vi "SetCheckedStatus.vi"(8 "error in (no error)":errorcluster, 9 "Checked":bool, 10 "MenuItem":refnum<class "MGI_MenuItem.lvclass">, 11 "Control in":refnum<class "MGI_Control.lvclass">) -> (0 "error out":errorcluster, 3 "Control out":refnum<class "MGI_Control.lvclass">)   [LabVIEW 2016, in "MGI_Control.lvclass"]
doc: "Sets the Checked Status.\n\nAuthored by Derek E. Trepanier\nsupport@mooregoodideas.com\nwww.mooregoodideas.com\n\nCopyright (c) 2012, Moore Good Ideas, Inc.\n\nAll rights reserved.\n\nRedistribution and use in source and binary forms, with or without modification, are permitted provided that the following conditions are met:\n\n * Redistributions of source code must retain the above copyright notice, this list of conditions and the following disclaimer.\n * Redistributions in binary form must reproduce the above copyright notice, this list of conditions and the following disclaimer in the documentation and/or other materials provided with the distribution.\n * Neither the name of Moore Good Ideas, Inc. nor the names of its contributors may be used to endorse or promote products derived from this software without specific prior written permission.\n\nTHIS SOFTWARE IS PROVIDED BY THE COPYRIGHT HOLDERS AND CONTRIBUTORS \"AS IS\" AND ANY EXPRESS OR IMPLIED WARRANTIES, INCLUDING, BUT NOT LIMITED TO, THE IMPLIED WARRANTIES OF MERCHANTABILITY AND FITNESS FOR A PARTICULAR PURPOSE ARE DISCLAIMED. IN NO EVENT SHALL THE COPYRIGHT OWNER OR CONTRIBUTORS BE LIABLE FOR ANY DIRECT, INDIRECT, INCIDENTAL, SPECIAL, EXEMPLARY, OR CONSEQUENTIAL DAMAGES (INCLUDING, BUT NOT LIMITED TO, PROCUREMENT OF SUBSTITUTE GOODS OR SERVICES; LOSS OF USE, DATA, OR PROFITS; OR BUSINESS INTERRUPTION) HOWEVER CAUSED AND ON ANY THEORY OF LIABILITY, WHETHER IN CONTRACT, STRICT LIABILITY, OR TORT (INCLUDING NEGLIGENCE OR OTHERWISE) ARISING IN ANY WAY OUT OF THE USE OF THIS SOFTWARE, EVEN IF ADVISED OF THE POSSIBILITY OF SUCH DAMAGE."
uses:
  <userlib>/_MGI/Menu Building/MenuTypes/Control/MGI_Control.lvclass
  <userlib>/_MGI/Menu Building/MenuItem/MGI_MenuItem.lvclass
  <userlib>/_MGI/Menu Building/MenuTypes/Control/MGI_Control.lvclass/MGI_Control.ctl
  <userlib>/_MGI/Menu Building/MenuItem/Read Full Tag.vi
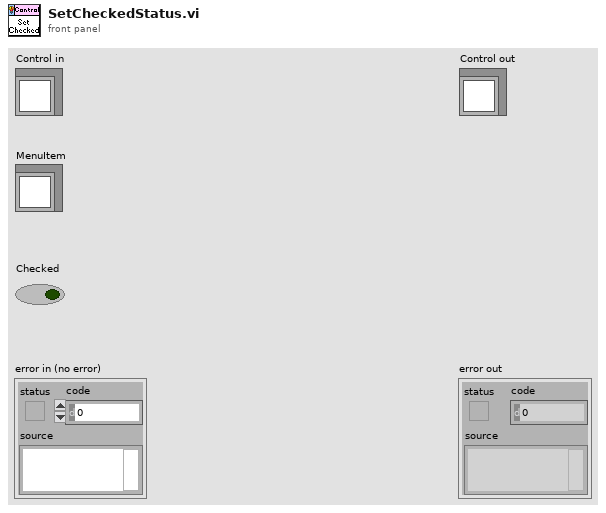
[diagram p1: front panel]
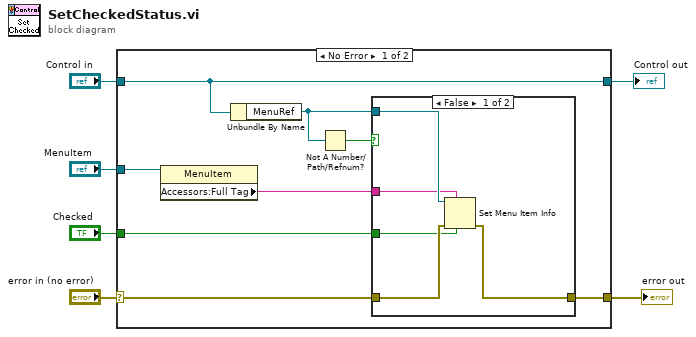
[diagram p0: block diagram]
diagram:
  n1 = case shown="No Error" "error in (no error)" {
    selector: "error in (no error)" -> [w8 w22]
    tunnel: "Control in" -> [w14 w21]
    tunnel: [w7 w22] -> w2
    tunnel: [w14 w21] -> w3
    tunnel: "MenuItem" -> [w11 _]
    tunnel: "Checked" -> [w9 _]
    frame No Error {
      n2 = property class="MenuItem"(reference=w11) -> ("Accessors:Full Tag"=w10:string)  [unwired: 1 in, 2 out]
      n3 = Unbundle By Name(w14) -> ("MenuRef"=w12:refnum<k9>)
      n4 = Not A Number/Path/Refnum?(number/path/refnum=w12) -> (NaN/Path/Refnum?=w13:bool)
      n5 = case shown="False" w13 {
        tunnel: w12 -> [w19 _]
        tunnel: w10 -> [w18 _]
        tunnel: w9 -> [w15 _]
        tunnel: w8 -> [w17 w20]
        tunnel: [w16 w20] -> w7
        frame False {
          n6 = Set Menu Item Info(6:w15, 7:w18, 8:w17, 11:w19) -> (0:w16:errorcluster)  [unwired: 3 in, 1 out]
        }
        frame True {
        }
      }
    }
    frame Error {
    }
  }
  "error out" <- w2
  "Control out" <- w3
